vi "test kalman filter.vi"() -> ()   [LabVIEW 2010]
uses:
  kalman pv state.ctl
panel:
  out "ticks":u32
  in  "RMS":u16 caption="noise rms"
  out "predict":T1
  out "in":T1
  out "meas":T1
  out "x meas":i32
  out "Waveform Chart":cluster{i32, i16}(graph)
  in  "n loops":i32=10000
  in  "n steps":i16=1000
  out "Kalman PV state out":T1
  in  "xmax":i16=1000
  in  "Kalman PV state":T1={"estimates"={"x"=0.0, "v"=41.0, "pxx"=0, "pxv"=0, "pvv"=0}, "model params"={"qxx"=1, "qxv"=2, "qvv"=4, "r"=100}}
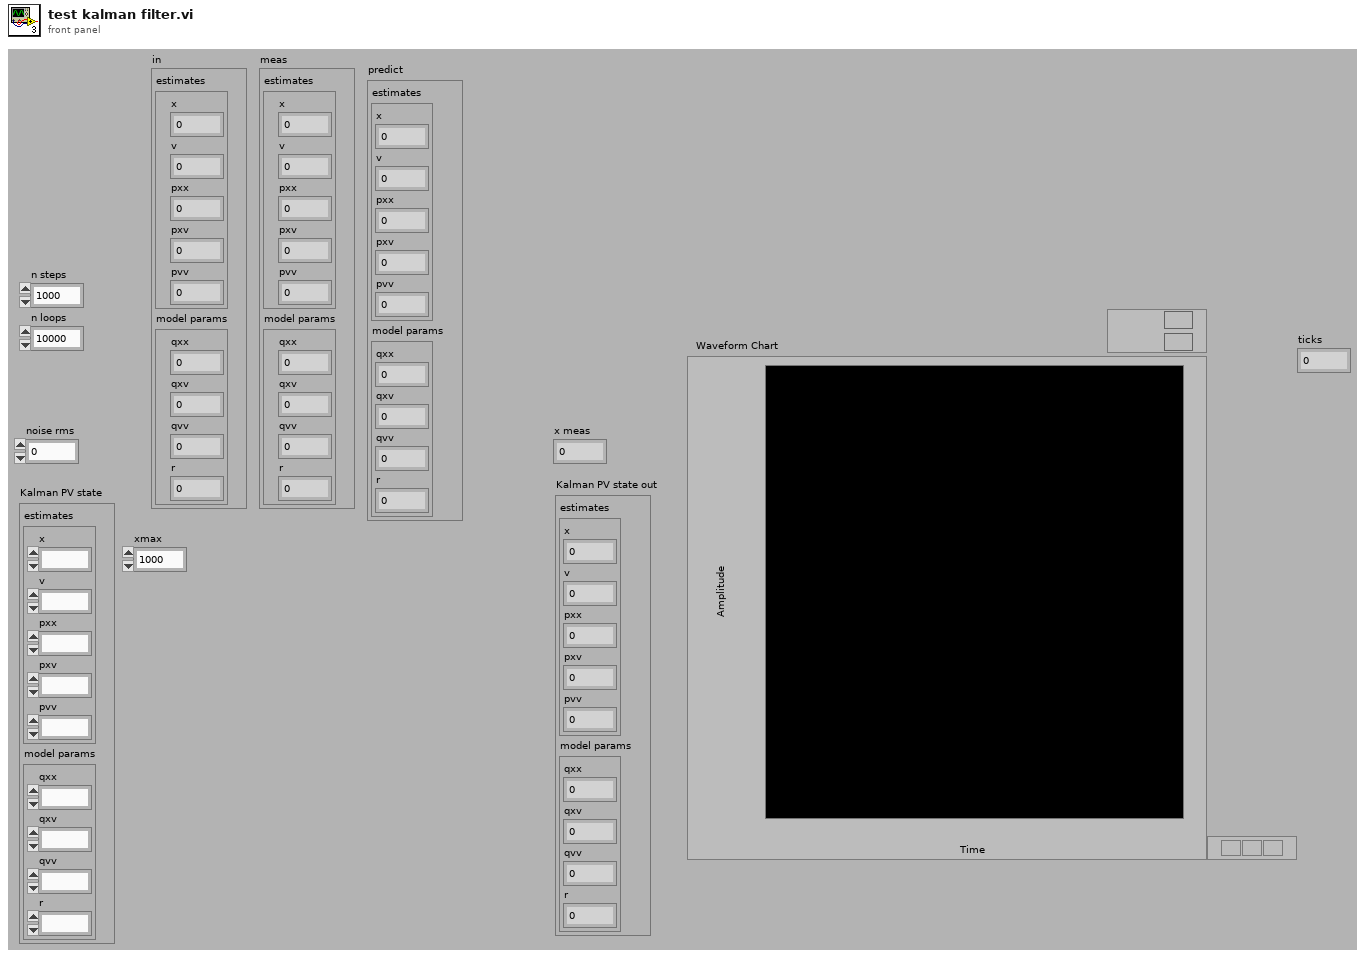
[diagram p1: front panel]
types:
  T1 = typedef "kalman pv state.ctl" = cluster{"estimates":cluster{"x":fxp<+/-,18,16>, "v":fxp<+/-,18,16>, "pxx":u16, "pxv":u16, "pvv":u16}, "model params":cluster{"qxx":u16, "qxv":u16, "qvv":u16, "r":u16}}
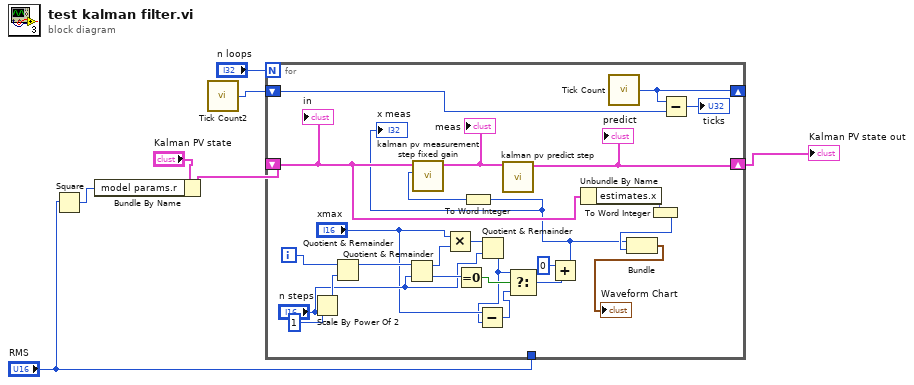
[diagram p0: block diagram]
diagram:
  n1 = Square(x="RMS") -> (x^2=w3:u16)
  n2 = Bundle By Name(cluster="Kalman PV state", "model params.r"=w3) -> (w4:T1)
  n3 = call "Tick Count2"() -> ("Tick Count(Ticks)"=w1:u32)
  n4 = for {
    N: "n loops" -> [_]
    shift-right: [w19] -> w5
    shift-left: w4 -> [w14]
    tunnel: "RMS" -> [_]
    shift-right: [w12] -> _
    shift-left: w1 -> [w11]
    i -> [w31]
    n5 = Scale By Power Of 2(n=1, x="n steps") -> (x*2^n=w29:i16)
    n6 = Quotient & Remainder(x=w31, y=w29) -> (x-y*floor(x/y)=w28:i32)  [unwired: 1 out]
    n7 = Quotient & Remainder(x=w28, y="n steps") -> (x-y*floor(x/y)=w26:i32, floor(x/y)=w27:i32)
    n8 = Multiply(x="xmax", y=w26) -> (x*y=w25:i32)
    n9 = Equal To 0?(x=w27) -> (x = 0?=w23:bool)
    n10 = Quotient & Remainder(x=w25, y="n steps") -> (floor(x/y)=w21:i32)  [unwired: 1 out]
    n11 = Subtract(x="xmax", y=w21) -> (x-y=w20:i32)
    n12 = Select(t=w21, s=w23, f=w20) -> (s? t:f=w17:i32)
    n13 = Add(x=0, y=w17) -> (x+y=w13:i32)
    "x meas" <- w13
    n14 = To Word Integer(number=w13) -> (16bit integer=w15:i16)
    n15 = call "kalman pv measurement step fixed gain.vi"("position measurement"=w15, "Kalman PV state"=w14) -> ("kalman pv state out"=w32:T1)  [unwired: 9 in]
    "meas" <- w32
    n16 = call "kalman pv predict step.vi"("Kalman PV state"=w32) -> ("Kalman PV state out"=w19:T1)  [unwired: 10 in]
    "predict" <- w19
    n17 = Unbundle By Name(w14) -> ("estimates.x"=w18:fxp<+/-,18,16>)
    n18 = call "Tick Count"() -> ("Tick Count(Ticks)"=w12:u32)
    n19 = To Word Integer(number=w18) -> (16bit integer=w16:i16)
    n20 = Bundle(w13, w16) -> (→"Waveform Chart":cluster{i32, i16})  [unwired: 1 in]
    n21 = Subtract(x=w12, y=w11) -> (x-y=→"ticks":u32)
    "in" <- w14
  }
  "Kalman PV state out" <- w5
